vi "CRYTest and Insert CRY6181 Signal Type.vi"(11 "Calibration In":T1 {"Calibration 2D"."Sens Curve"."Z data" items=["dB", "Lin"]; "Calibration 2D"."Sens Curve"."X data" items=["dB", "Lin"]; "Calibration 2D"."Sens Curve"."Y data" items=["dB", "Lin"]; "Calibration 2D"."Sens Curve"."Z dB ref" format="%.1f"; "Calibration 2D"."Sens Curve"."Z axis" items=["Log", "Lin"]; "Calibration 2D"."Sens Curve"."X dB ref" format="%.1f"; "Calibration 2D"."Sens Curve"."X axis" items=["Log", "Lin"]; "Calibration 2D"."Sens Curve"."Y axis" items=["Log", "Lin"]; "Calibration 2D"."Sens Curve"."Y dB ref" format="%.1f"; "Calibration 2D"."Sens Curve"."Curve"."z" format="%.2f"; "Calibration 2D"."Sens Curve"."Curve"."y" format="%.2f"; "Calibration 2D"."Sens Curve"."Curve"."x" format="%.2f"; "Calibration 2D"."EQ Curve"."Z data" items=["dB", "Lin"]; "Calibration 2D"."EQ Curve"."X data" items=["dB", "Lin"]; "Calibration 2D"."EQ Curve"."Y data" items=["dB", "Lin"]; "Calibration 2D"."EQ Curve"."Z dB ref" format="%.1f"; "Calibration 2D"."EQ Curve"."Z axis" items=["Log", "Lin"]; "Calibration 2D"."EQ Curve"."X dB ref" format="%.1f"; "Calibration 2D"."EQ Curve"."X axis" items=["Log", "Lin"]; "Calibration 2D"."EQ Curve"."Y axis" items=["Log", "Lin"]; "Calibration 2D"."EQ Curve"."Y dB ref" format="%.1f"; "Calibration 2D"."EQ Curve"."Curve"."z" format="%.2f"; "Calibration 2D"."EQ Curve"."Curve"."y" format="%.2f"; "Calibration 2D"."EQ Curve"."Curve"."x" format="%.2f"; "Calibration 2D"."Corr Curve"."Z data" items=["dB", "Lin"]; "Calibration 2D"."Corr Curve"."X data" items=["dB", "Lin"]; "Calibration 2D"."Corr Curve"."Y data" items=["dB", "Lin"]; "Calibration 2D"."Corr Curve"."Z dB ref" format="%.1f"; "Calibration 2D"."Corr Curve"."Z axis" items=["Log", "Lin"]; "Calibration 2D"."Corr Curve"."X dB ref" format="%.1f"; "Calibration 2D"."Corr Curve"."X axis" items=["Log", "Lin"]; "Calibration 2D"."Corr Curve"."Y axis" items=["Log", "Lin"]; "Calibration 2D"."Corr Curve"."Y dB ref" format="%.1f"; "Calibration 2D"."Corr Curve"."Curve"."z" format="%.2f"; "Calibration 2D"."Corr Curve"."Curve"."y" format="%.2f"; "Calibration 2D"."Corr Curve"."Curve"."x" format="%.2f"; "Calibration 2D"."Calibration"."EQ Step size" items=["R10", "R20", "R40", "R80", "User"]; "Calibration 2D"."Calibration"."Corr Step size" items=["R10", "R20", "R40", "R80", "User"]}) -> (0 "Inserted signal type":bool, 3 "Calibration out":T1 {"Calibration 2D"."Sens Curve"."Z data" items=["dB", "Lin"]; "Calibration 2D"."Sens Curve"."X data" items=["dB", "Lin"]; "Calibration 2D"."Sens Curve"."Y data" items=["dB", "Lin"]; "Calibration 2D"."Sens Curve"."Z dB ref" format="%.1f"; "Calibration 2D"."Sens Curve"."Z axis" items=["Log", "Lin"]; "Calibration 2D"."Sens Curve"."X dB ref" format="%.1f"; "Calibration 2D"."Sens Curve"."X axis" items=["Log", "Lin"]; "Calibration 2D"."Sens Curve"."Y axis" items=["Log", "Lin"]; "Calibration 2D"."Sens Curve"."Y dB ref" format="%.1f"; "Calibration 2D"."Sens Curve"."Curve"."z" format="%.2f"; "Calibration 2D"."Sens Curve"."Curve"."y" format="%.2f"; "Calibration 2D"."Sens Curve"."Curve"."x" format="%.2f"; "Calibration 2D"."EQ Curve"."Z data" items=["dB", "Lin"]; "Calibration 2D"."EQ Curve"."X data" items=["dB", "Lin"]; "Calibration 2D"."EQ Curve"."Y data" items=["dB", "Lin"]; "Calibration 2D"."EQ Curve"."Z dB ref" format="%.1f"; "Calibration 2D"."EQ Curve"."Z axis" items=["Log", "Lin"]; "Calibration 2D"."EQ Curve"."X dB ref" format="%.1f"; "Calibration 2D"."EQ Curve"."X axis" items=["Log", "Lin"]; "Calibration 2D"."EQ Curve"."Y axis" items=["Log", "Lin"]; "Calibration 2D"."EQ Curve"."Y dB ref" format="%.1f"; "Calibration 2D"."EQ Curve"."Curve"."z" format="%.2f"; "Calibration 2D"."EQ Curve"."Curve"."y" format="%.2f"; "Calibration 2D"."EQ Curve"."Curve"."x" format="%.2f"; "Calibration 2D"."Corr Curve"."Z data" items=["dB", "Lin"]; "Calibration 2D"."Corr Curve"."X data" items=["dB", "Lin"]; "Calibration 2D"."Corr Curve"."Y data" items=["dB", "Lin"]; "Calibration 2D"."Corr Curve"."Z dB ref" format="%.1f"; "Calibration 2D"."Corr Curve"."Z axis" items=["Log", "Lin"]; "Calibration 2D"."Corr Curve"."X dB ref" format="%.1f"; "Calibration 2D"."Corr Curve"."X axis" items=["Log", "Lin"]; "Calibration 2D"."Corr Curve"."Y axis" items=["Log", "Lin"]; "Calibration 2D"."Corr Curve"."Y dB ref" format="%.1f"; "Calibration 2D"."Corr Curve"."Curve"."z" format="%.2f"; "Calibration 2D"."Corr Curve"."Curve"."y" format="%.2f"; "Calibration 2D"."Corr Curve"."Curve"."x" format="%.2f"; "Calibration 2D"."Calibration"."EQ Step size" items=["R10", "R20", "R40", "R80", "User"]; "Calibration 2D"."Calibration"."Corr Step size" items=["R10", "R20", "R40", "R80", "User"]})   [LabVIEW 2013]
uses:
  Typedef Control/CRYCalibration All Cluster.ctl
  Typedef Control/CRYCalibration 2DCluster.ctl
  Typedef Control/CRYCalibration Cluster.ctl
  Typedef Control/CRYData Cluster.ctl
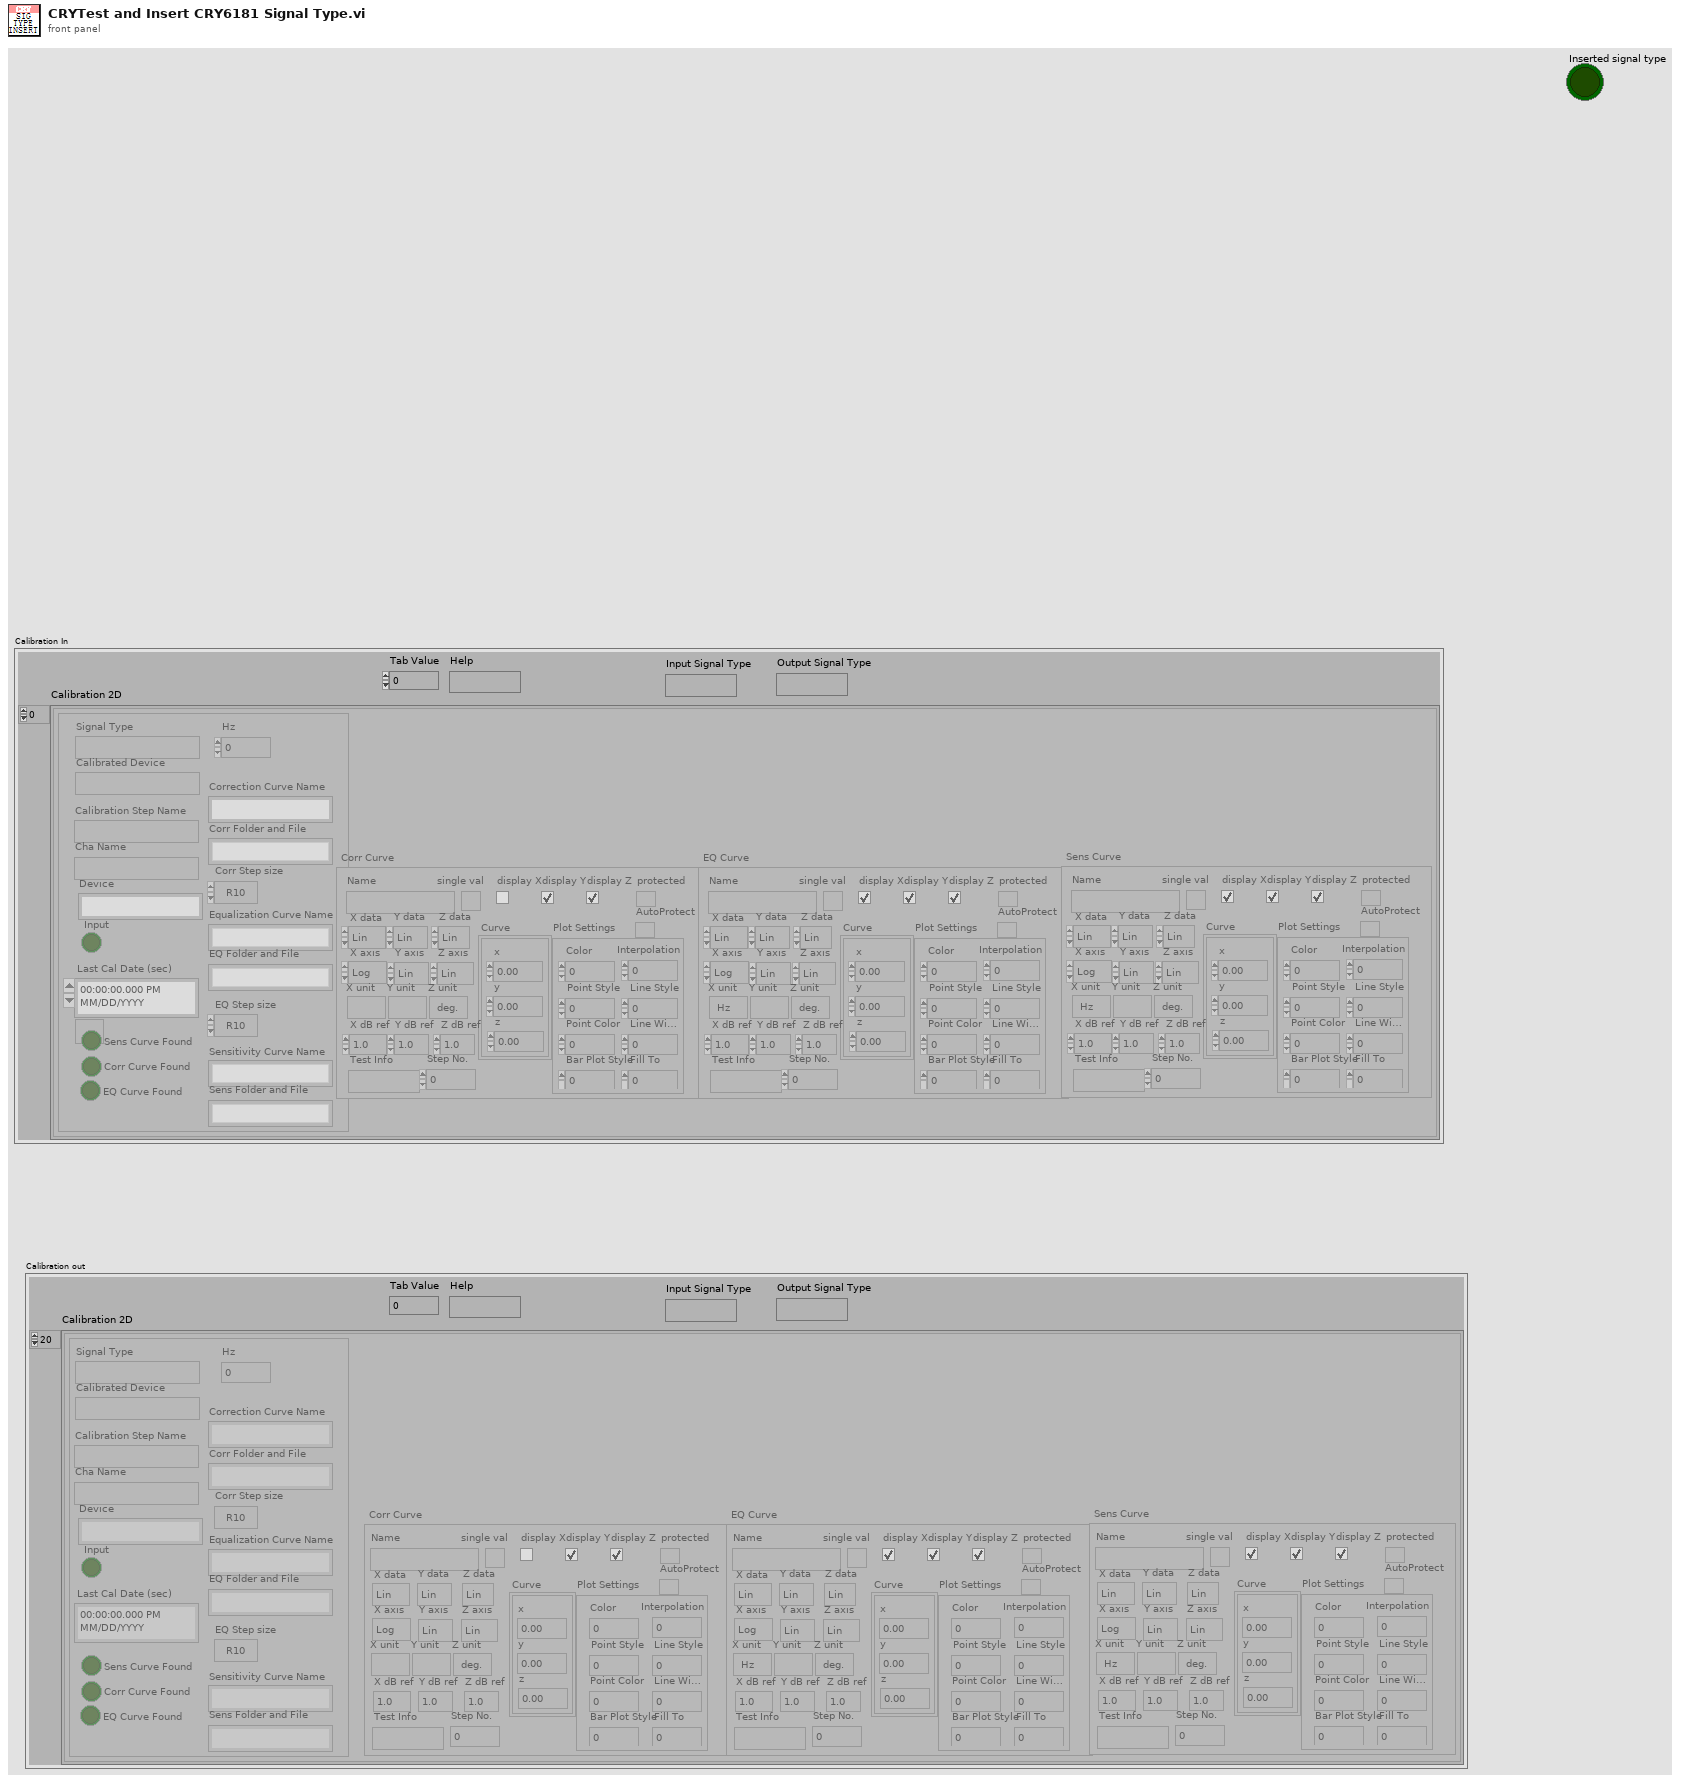
[diagram p1: front panel]
types:
  T1 = typedef "CRYCalibration All Cluster.ctl" = cluster{"Calibration 2D":T2[], "Help":string, "Tab Value":i32, "Input Signal Type":string, "Output Signal Type":string}
  T2 = typedef "CRYCalibration 2DCluster.ctl" = cluster{"Calibration":T3, "Corr Curve":T4, "EQ Curve":T4, "Sens Curve":T4}
  T3 = typedef "CRYCalibration Cluster.ctl" = cluster{"Calibration Step Name":string, "Device":string, "Correction Curve Name":string, "Equalization Curve Name":string, "Sensitivity Curve Name":string, "Corr Folder and File":string, "EQ Folder and File":string, "Sens Folder and File":string, "Corr Step size":u16, "EQ Step size":u16, "Input":bool, "Last Cal Date (sec)":timestamp, "Cha Name":string, "Corr Curve Found":bool, "EQ Curve Found":bool, "Sens Curve Found":bool, "Signal Type":string, "Calibrated Device":string, "Hz":u32}
  T4 = typedef "CRYData Cluster.ctl" = cluster{"Name":string, "Curve":cluster{"x":dbl, "y":dbl, "z":dbl}[], "X data":u16, "Y data":u16, "Z data":u16, "X axis":u16, "Y axis":u16, "Z axis":u16, "X unit":string, "Y unit":string, "Z unit":string, "X dB ref":dbl, "Y dB ref":dbl, "Z dB ref":dbl, "single val":bool, "protected":bool, "display X":bool, "display Y":bool, "display Z":bool, "Test Info":string, "Step No.":i32, "Plot Settings":cluster{"Color":u32, "Interpolation":u8, "Point Style":u8, "Line Style":u8, "Point Color":u32, "Line Width":u8, "Bar Plot Style":u8, "Fill To":i16}, "AutoProtect":bool}
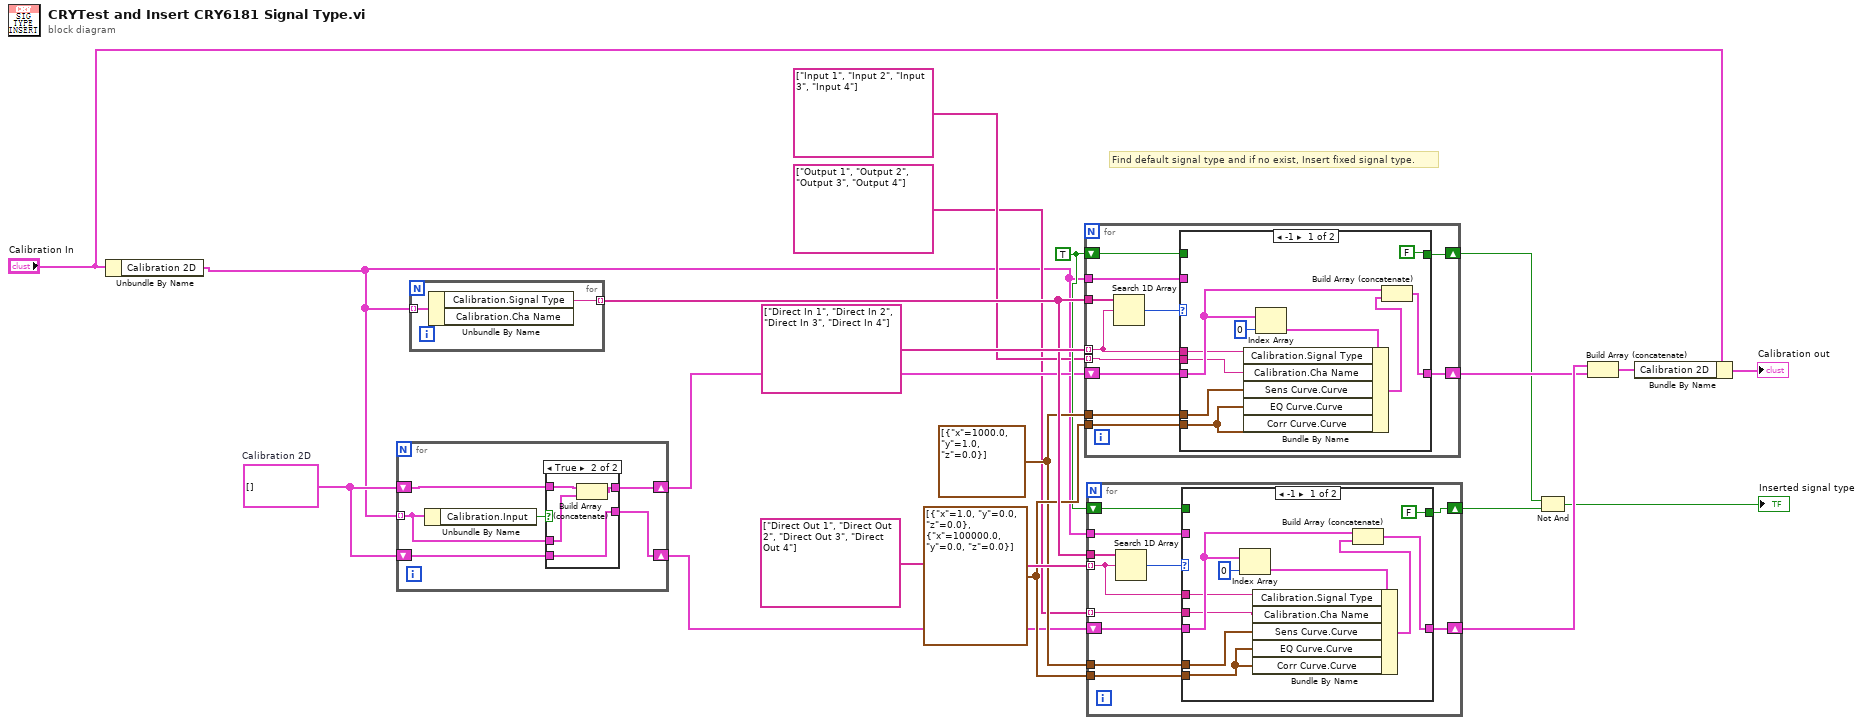
[diagram p0: block diagram]
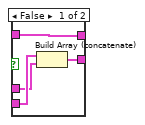
[diagram p2: hidden frame]
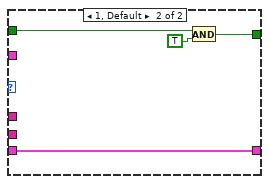
[diagram p3: hidden frame]
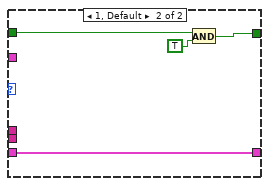
[diagram p4: hidden frame]
diagram:
  w15 = cluster{"x":dbl, "y":dbl, "z":dbl}[] [{"x"=1.0, "y"=0.0, "z"=0.0}, {"x"=100000.0, "y"=0.0, "z"=0.0}] ("EQ Curve.Curve")
  w14 = cluster{"x":dbl, "y":dbl, "z":dbl}[] [{"x"=1000.0, "y"=1.0, "z"=0.0}] ("Sens Curve.Curve")
  w9 = T2[] []  # Calibration 2D
  w11 = TRUE
  # "Find default signal type and if no exist, Insert fixed signal type."
  n1 = Unbundle By Name("Calibration In") -> ("Calibration 2D"=w4:T2[])
  n2 = for {
    tunnel: w4 -> [w25] mode=indexing
    shift-right: [w21] -> w8
    shift-left: w9 -> [w22]
    shift-right: [w23] -> w10
    shift-left: w9 -> [w24]
    n3 = Unbundle By Name(w25) -> ("Calibration.Input"=w26:bool)
    n4 = case shown="True" w26 {
      tunnel: w25 -> [w29 w33]
      tunnel: w24 -> [w27 w34]
      tunnel: [w27 w32] -> w23
      tunnel: w22 -> [w30 w31]
      tunnel: [w28 w31] -> w21
      frame False {
        n5 = Build Array (concatenate)(w30, w29) -> (w28:T2[])
      }
      frame True {
        n6 = Build Array (concatenate)(w34, w33) -> (w32:T2[])
      }
    }
  }
  n7 = for {
    tunnel: w4 -> [w36] mode=indexing
    tunnel: [w35] -> w18 mode=indexing
    n8 = Unbundle By Name(w36) -> ("Calibration.Signal Type"=w35:string)  [unwired: 1 out]
  }
  n9 = for {
    tunnel: string[] ["Direct In 1", "Direct In 2", "Direct In 3", "Direct In 4"] -> [w45] mode=indexing
    tunnel: w18 -> [w46]
    tunnel: w4 -> [w43]
    shift-right: [w47] -> w16
    shift-left: w10 -> [w42]
    shift-right: [w40] -> w13
    shift-left: w11 -> [w41]
    tunnel: w14 -> [w39]
    tunnel: w15 -> [w38]
    tunnel: string[] ["Input 1", "Input 2", "Input 3", "Input 4"] -> [w37] mode=indexing
    n10 = Search 1D Array(1D array=w46, element=w45) -> (index of element=w44:i32)  [unwired: 1 in]
    n11 = case shown="-1" w44 {
      tunnel: [w55 w58] -> w47
      tunnel: w45 -> [w52 _]
      tunnel: w43 -> [_ _]
      tunnel: w42 -> [w56 w58]
      tunnel: w41 -> [_ w60]
      tunnel: [FALSE w59] -> w40
      tunnel: w39 -> [w50 _]
      tunnel: w38 -> [w49 _]
      tunnel: w37 -> [w51 _]
      frame -1 {
        n12 = Index Array(array=w56, index=0) -> (element=w54:T2)
        n13 = Bundle By Name(cluster=w54, "Calibration.Signal Type"=w52, "Calibration.Cha Name"=w51, "Sens Curve.Curve"=w50, "EQ Curve.Curve"=w49, "Corr Curve.Curve"=w49) -> (w53:T2)
        n14 = Build Array (concatenate)(w56, w53) -> (w55:T2[])
      }
      frame 1, Default {
        n15 = And(x=w60, y=TRUE) -> (x .and. y?=w59:bool)
      }
    }
  }
  n16 = for {
    tunnel: string[] ["Direct Out 1", "Direct Out 2", "Direct Out 3", "Direct Out 4"] -> [w70] mode=indexing
    tunnel: w18 -> [w71]
    tunnel: w4 -> [w68]
    shift-right: [w72] -> w17
    shift-left: w8 -> [w67]
    shift-right: [w65] -> w12
    shift-left: w11 -> [w66]
    tunnel: w15 -> [w64]
    tunnel: w14 -> [w63]
    tunnel: string[] ["Output 1", "Output 2", "Output 3", "Output 4"] -> [w62] mode=indexing
    n17 = Search 1D Array(1D array=w71, element=w70) -> (index of element=w69:i32)  [unwired: 1 in]
    n18 = case shown="-1" w69 {
      tunnel: [w79 w83] -> w72
      tunnel: w70 -> [w76 _]
      tunnel: w68 -> [_ _]
      tunnel: w67 -> [w80 w83]
      tunnel: w66 -> [_ w85]
      tunnel: [FALSE w84] -> w65
      tunnel: w64 -> [w73 _]
      tunnel: w63 -> [w74 _]
      tunnel: w62 -> [w75 _]
      frame -1 {
        n19 = Index Array(array=w80, index=0) -> (element=w77:T2)
        n20 = Bundle By Name(cluster=w77, "Calibration.Signal Type"=w76, "Calibration.Cha Name"=w75, "Sens Curve.Curve"=w74, "EQ Curve.Curve"=w73, "Corr Curve.Curve"=w73) -> (w78:T2)
        n21 = Build Array (concatenate)(w80, w78) -> (w79:T2[])
      }
      frame 1, Default {
        n22 = And(x=w85, y=TRUE) -> (x .and. y?=w84:bool)
      }
    }
  }
  n23 = Not And(1:w12, 2:w13) -> (0:→"Inserted signal type":bool)
  n24 = Build Array (concatenate)(w17, w16) -> (w1:T2[])
  n25 = Bundle By Name(cluster="Calibration In", "Calibration 2D"=w1) -> (→"Calibration out":T1)
